vi "CustomTimer.vi"(4 "error in (no error)":errorcluster, 5 "Clear":bool, 7 "Start":bool) -> (0 "error out":errorcluster, 1 "timeText":string, 2 "secondText":string, 3 "elapsedSecond":i32)   [LabVIEW 2015]
doc: "计时器\nsuspend:true 计时\n false 暂停\nelapsedSecond:所用的时间"
panel:
  out "preElapsed":i32
  in  "count?":bool
  out "Start":u32
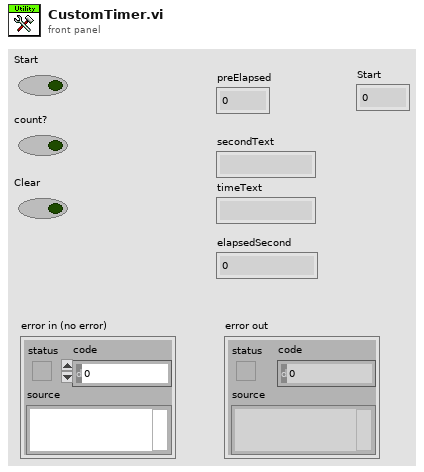
[diagram p1: front panel]
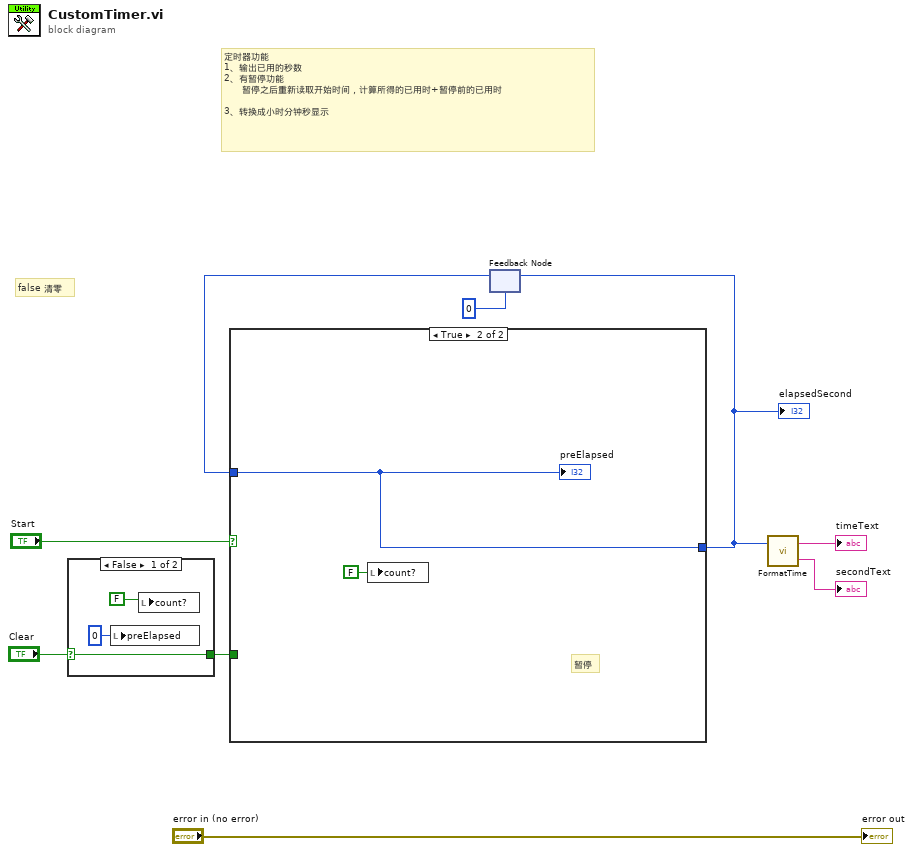
[diagram p0: block diagram]
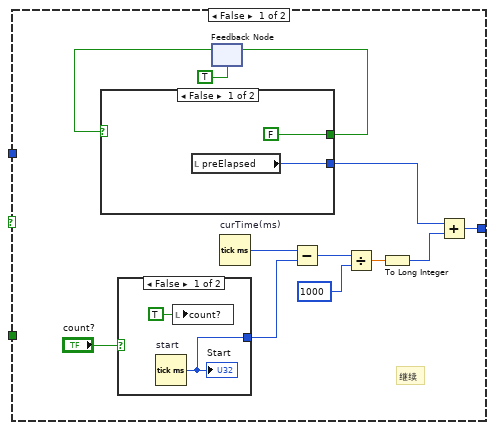
[diagram p3: hidden frame]
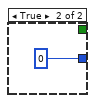
[diagram p4: hidden frame]
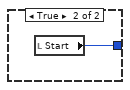
[diagram p5: hidden frame]
diagram:
  # "false 清零"
  # "定时器功能 \n1、输出已用的秒数\n2、有暂停功能\n      暂停之后重新读取开始时间，计算所得的已用时+暂停前的已用时\n\n3、转换成小时分钟秒显示"
  n1 = case shown="False" "Clear" {
    selector: "Clear" -> [w12 w13]
    tunnel: [w12 w13] -> w1
    frame False {
      n2 = local write "preElapsed"(0 ("preElapsed")) -> ()
      n3 = local write "count?"(FALSE ("count?")) -> ()
    }
    frame True {
    }
  }
  n4 = feedback #1(0) -> (w5:i32)
  n5 = case shown="True" "Start" {
    tunnel: [w19 w32] -> w4
    tunnel: w5 -> [_ w32]
    tunnel: w1 -> [_ _]
    frame False {
      # "继续"
      n6 = case shown="False" "count?" {
        tunnel: [w30 w31] -> w22
        frame False {
          n7 = Tick Count (ms) "start"() -> (millisecond timer value=w30:u32)
          "Start" <- w30
          n8 = local write "count?"(TRUE ("count?")) -> ()
        }
        frame True {
          n9 = local read "Start"() -> (w31:u32)
        }
      }
      n10 = feedback #2(TRUE ("count?")) -> (w17:bool)
      n11 = case shown="False" w17 {
        tunnel: [FALSE ("count?") _] -> w16
        tunnel: [w26 0 ("preElapsed")] -> w15
        frame False {
          n12 = local read "preElapsed"() -> (w26:i32)
        }
        frame True {
        }
      }
      n13 = feedback-in #2(w16) -> ()
      n14 = Tick Count (ms) "curTime(ms)"() -> (millisecond timer value=w25:u32)
      n15 = Subtract(x=w25, y=w22) -> (x-y=w24:u32)
      n16 = Divide(x=w24, y=u32 1000) -> (x/y=w21:dbl)
      n17 = To Long Integer(number=w21) -> (32bit integer=w20:i32)
      n18 = Add(x=w15, y=w20) -> (x+y=w19:i32)
    }
    frame True {
      # "暂停"
      n19 = local write "count?"(FALSE ("count?")) -> ()
      "preElapsed" <- w32
    }
  }
  "elapsedSecond" <- w4
  n20 = feedback-in #1(w4) -> ()
  n21 = call "FormatTime.vi"("secondNum"=w4) -> ("secondText"=→"secondText":string, "timeText"=→"timeText":string)  [unwired: 1 in]
  "error out" <- "error in (no error)"
